vi "CRC.vi"(11 "Sequence Config in":refnum<class "Sequence Config.lvclass">) -> (2 "CRC":u32, 3 "Sequence Config out":refnum<class "Sequence Config.lvclass">)   [LabVIEW 2020, in "VolatusSeqConfig.lvlib" / "Sequence Config.lvclass"]
uses:
  Sequence Config.lvclass
  Sequence Config.lvclass/Sequence Config.ctl
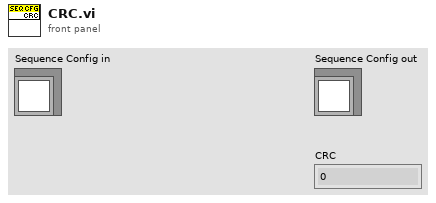
[diagram p1: front panel]
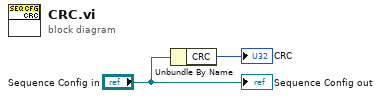
[diagram p0: block diagram]
diagram:
  n1 = Unbundle By Name("Sequence Config in") -> ("CRC"=→"CRC":u32)
  "Sequence Config out" <- "Sequence Config in"
